vi "TCP Router Worker.vi"(7 "Name(\"\" to use uuid)":string="CSM-Module") -> ()   [LabVIEW 2020]
uses:
  <userlib>/_NEVSTOP/Communicable State Machine(CSM)/_Support/Priority Queue/Priority Queue.lvclass/Priority Queue.ctl
  4e85c3fb-ef85-4e26-a42c-c5beb394b70a.vi
  3806dceb-3f37-4f57-9f18-971811feca89.vi
  9016553c-cc0c-45c9-a77e-ad45dca8b9f9.vi
  29aca12e-f851-4e59-a4c5-05d041862115.vi
  20f56057-ddbc-4e16-b502-c2d75e71b705.vi
  <userlib>/_NEVSTOP/Communicable State Machine(CSM)/_Support/Process/CSMP-Async Call.vi
  <userlib>/_NEVSTOP/Communicable State Machine(CSM)/_Support/GlobalEvent/GEvt-Generate Status Log.vi
  <userlib>/_NEVSTOP/Communicable State Machine(CSM)/_Support/Process/CSMP-Broadcast.vi
  <userlib>/_NEVSTOP/Communicable State Machine(CSM)/_Support/GlobalEvent/GEvt-Generate Interrupt Log.vi
  <userlib>/_NEVSTOP/Communicable State Machine(CSM)/_Support/Process/CSMP-Register Status.vi
  <userlib>/_NEVSTOP/Communicable State Machine(CSM)/_Support/GlobalEvent/GEvt-Generate Register Log.vi
  <userlib>/_NEVSTOP/Communicable State Machine(CSM)/_Support/Process/CSMP-Unregister Status.vi
  <userlib>/_NEVSTOP/Communicable State Machine(CSM)/_Support/GlobalEvent/GEvt-Generate Unregister Log.vi
  <userlib>/_NEVSTOP/Communicable State Machine(CSM)/_Support/Process/CSMP-Sync Call.vi
  <userlib>/_NEVSTOP/Communicable State Machine(CSM)/_Support/CSMQ/_CSMObj-Unlock.vi
  <userlib>/_NEVSTOP/Communicable State Machine(CSM)/_Support/Process/CSMP-PostPostMsg.vi
  <userlib>/_NEVSTOP/Communicable State Machine(CSM)/_Support/Process/CSMP-PostSendMsg.vi
  <userlib>/_NEVSTOP/Communicable State Machine(CSM)/_Support/CSMQ/_CSMObj-Lock State.vi
  <userlib>/_NEVSTOP/Communicable State Machine(CSM)/_Support/Common/Splite Reason String Part.vi
  <userlib>/_NEVSTOP/Communicable State Machine(CSM)/_Support/Common/Trim Single line Text.vi
  <userlib>/_NEVSTOP/Communicable State Machine(CSM)/_Support/CSMQ/_CSMOFGV Release.vi
  <userlib>/_NEVSTOP/Communicable State Machine(CSM)/_Support/Common/Remove Comments from Line.vi
  <userlib>/_NEVSTOP/Communicable State Machine(CSM)/_Support/Common/Splite Single-line Message.vi
  <userlib>/_NEVSTOP/Communicable State Machine(CSM)/_Support/Common/Parse Next Single-line State.vi
  <userlib>/_NEVSTOP/Communicable State Machine(CSM)/_Support/CSMQ/_CSMOFGV Dequeue.vi
  <userlib>/_NEVSTOP/Communicable State Machine(CSM)/_Support/CSMQ/_CSMObj-Log Error if in a Remote Session.vi
  <userlib>/_NEVSTOP/Communicable State Machine(CSM)/_Support/GlobalEvent/GEvt-Generate State Change Log.vi
  <userlib>/_NEVSTOP/Communicable State Machine(CSM)/_Support/GlobalEvent/GEvt-Generate Remaining States Log.vi
  <userlib>/_NEVSTOP/Communicable State Machine(CSM)/_Support/GlobalEvent/GEvt-Generate Module Destroyed Log.vi
  <userlib>/_NEVSTOP/Communicable State Machine(CSM)/_Support/GlobalEvent/GEvt-Generate Complete Log.vi
  <userlib>/_NEVSTOP/Communicable State Machine(CSM)/_Support/GlobalEvent/GEvt-Generate Module Created Log.vi
  <userlib>/_NEVSTOP/Communicable State Machine(CSM)/_Support/GlobalEvent/Cache-GEvt Filter Object.vi
  <userlib>/_NEVSTOP/Communicable State Machine(CSM)/AdvanceAPI/CSM - Revert Arguments-Safe String.vi
  <userlib>/_NEVSTOP/Communicable State Machine(CSM)/AdvanceAPI/CSM - Make String Arguments Safe.vi
  <userlib>/_NEVSTOP/Communicable State Machine(CSM)/AdvanceAPI/CSM - Break Down Multiple States String.vi
  <userlib>/_NEVSTOP/Communicable State Machine(CSM)/AdvanceAPI/CSM - Compact Multiple States.vi
  <userlib>/_NEVSTOP/Communicable State Machine(CSM)/addons/API-String-Arugments-Support/_Support/Query Data as API String Arguments(variant).vi
  <userlib>/_NEVSTOP/Communicable State Machine(CSM)/_Support/CSMQ/_Obtain CSM Data Queue.vi
  <userlib>/_NEVSTOP/Communicable State Machine(CSM)/_Support/Priority Queue/Release Priority Queue.vi
  <userlib>/_NEVSTOP/Communicable State Machine(CSM)/_Support/CSMQ/_CSMObj-Message Check.vi
  <userlib>/_NEVSTOP/Communicable State Machine(CSM)/_Support/CSMQ/_CSMObj-Enqueue Cross-Module Message.vi
  <userlib>/_NEVSTOP/Communicable State Machine(CSM)/_Support/CSMQ/_CSMOFGV Get.vi
  <userlib>/_NEVSTOP/Communicable State Machine(CSM)/_Support/GlobalEvent/GEvt-Generate with Rule Check.vi
  <userlib>/_NEVSTOP/Communicable State Machine(CSM)/_Support/FGV-BroadcastRegistry/Cache-Broadcast Registry Search Result.vi
  <userlib>/_NEVSTOP/Communicable State Machine(CSM)/_Support/Common/Hex Str to U8 Data.vi
  <userlib>/_NEVSTOP/Communicable State Machine(CSM)/_Support/Common/Concatenate State with Arguments.vi
  <userlib>/_NEVSTOP/Communicable State Machine(CSM)/_Support/Common/U8 Data to Hex Str.vi
  <userlib>/_NEVSTOP/Communicable State Machine(CSM)/_Support/Priority Queue/Dequeue Element.vi
  <userlib>/_NEVSTOP/Communicable State Machine(CSM)/AdvanceAPI/CSM - Keywords.vi
  <userlib>/_NEVSTOP/Communicable State Machine(CSM)/_Support/Priority Queue/Obtain Priority Queue.vi
  <userlib>/_NEVSTOP/Communicable State Machine(CSM)/_Support/Priority Queue/Enqueue Element.vi
  <userlib>/_NEVSTOP/Communicable State Machine(CSM)/Utility/Trim Both Whitespace.vi
  <userlib>/_NEVSTOP/Communicable State Machine(CSM)/_Support/GlobalEvent/FGV-GlobalEventRef.vi
  <userlib>/_NEVSTOP/Communicable State Machine(CSM)/_Support/GlobalEvent/global-GEvnt Filter Change Flag.vi
  <userlib>/_NEVSTOP/Communicable State Machine(CSM)/_Support/GlobalEvent/FGV-GEvt Filter Obj.vi
  <userlib>/_NEVSTOP/Communicable State Machine(CSM)/_Support/CSMQ/_CSMOFGV Obtain.vi
  <userlib>/_NEVSTOP/Communicable State Machine(CSM)/_Support/GlobalEvent/LogFilter/LogFilter - Check.vi
  <userlib>/_NEVSTOP/Communicable State Machine(CSM)/Utility/Build Internal State String.vi
  <userlib>/_NEVSTOP/Communicable State Machine(CSM)/_Support/CSMQ/_CSMOFGV.vi
  <userlib>/_NEVSTOP/Communicable State Machine(CSM)/_Support/Error/CSM Not Allowed Message.vi
  <userlib>/_NEVSTOP/Communicable State Machine(CSM)/_Support/GlobalEvent/FGV-StatusChangeEventRef.vi
  <userlib>/_NEVSTOP/Communicable State Machine(CSM)/_Support/FGV-BroadcastRegistry/global-CSMQ FGV Change Flag.vi
  <userlib>/_NEVSTOP/Communicable State Machine(CSM)/_Support/FGV-BroadcastRegistry/global-Broadcast Cache Change Flag.vi
  <userlib>/_NEVSTOP/Communicable State Machine(CSM)/_Support/BroadcastRegistry/HelperVI/Broadcast Item Key.vi
  <userlib>/_NEVSTOP/Communicable State Machine(CSM)/_Support/FGV-BroadcastRegistry/FGV-BroadcastRegistry.vi
  <userlib>/_NEVSTOP/Communicable State Machine(CSM)/_Support/Message/Parse Register Message.vi
  <userlib>/_NEVSTOP/Communicable State Machine(CSM)/_Support/CSMQ/_CSMObj-Add Internal Registry Rule.vi
  <userlib>/_NEVSTOP/Communicable State Machine(CSM)/_Support/Message/Parse Unregister Message.vi
  <userlib>/_NEVSTOP/Communicable State Machine(CSM)/_Support/CSMQ/_CSMObj-Unregister Internal Registry Rules.vi
  <userlib>/_NEVSTOP/Communicable State Machine(CSM)/addons/API-String-Arugments-Support/_Support/Data To SingleElementsArray_with_itself_csm.vi
  <userlib>/_NEVSTOP/Communicable State Machine(CSM)/addons/API-String-Arugments-Support/_Support/Data To API String Arguments.vi
  <userlib>/_NEVSTOP/Communicable State Machine(CSM)/addons/API-String-Arugments-Support/_Support/Convert API String Arguments to Data(variant).vi
  <userlib>/_NEVSTOP/Communicable State Machine(CSM)/_Support/Error/CSM No Target Error.vi
  <userlib>/_NEVSTOP/Communicable State Machine(CSM)/_Support/Priority Queue/Priority Queue.lvclass
  <userlib>/_NEVSTOP/Communicable State Machine(CSM)/Communicable State Machine.lvlib
  <userlib>/_NEVSTOP/Communicable State Machine(CSM)/_csmHelper/API with lvcsm Support/CSM-Helper API with lvcsm Support.lvlib
panel:
  out "Error Occurred":errorcluster
  out "State History":string
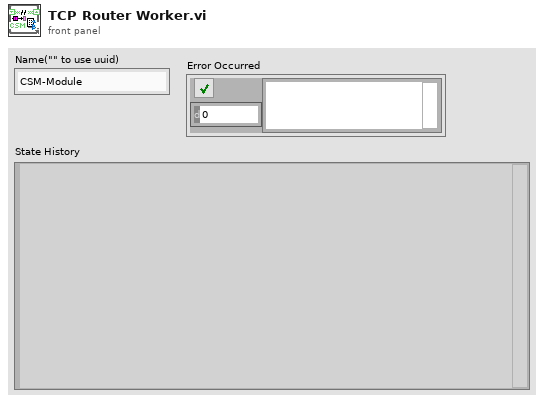
[diagram p1: front panel]
types:
  T1 = enum32{"Invalid", "Standard", "Closed", "Hidden", "Minimized", "Maximized"}
  T2 = enum32{"invalid app kind", "Development System", "Run Time System", "Student Edition", "Embedded LabVIEW", "Evaluation", "Custom"}
  T3 = typedef "Communicable State Machine.lvlib/_CSM_Response Source Message.ctl" = cluster{"‘State":string, "’Arguments":string, "’Error":errorcluster}
  T4 = cluster{"Current VI Reference":refnum<vi>, "Close Panel on Exit?":bool}
  T5 = cluster{"Core":cluster{"Current VI Reference":refnum<vi>, "Close Panel on Exit?":bool}, "Your Boolean data":bool, "Your string data":string}
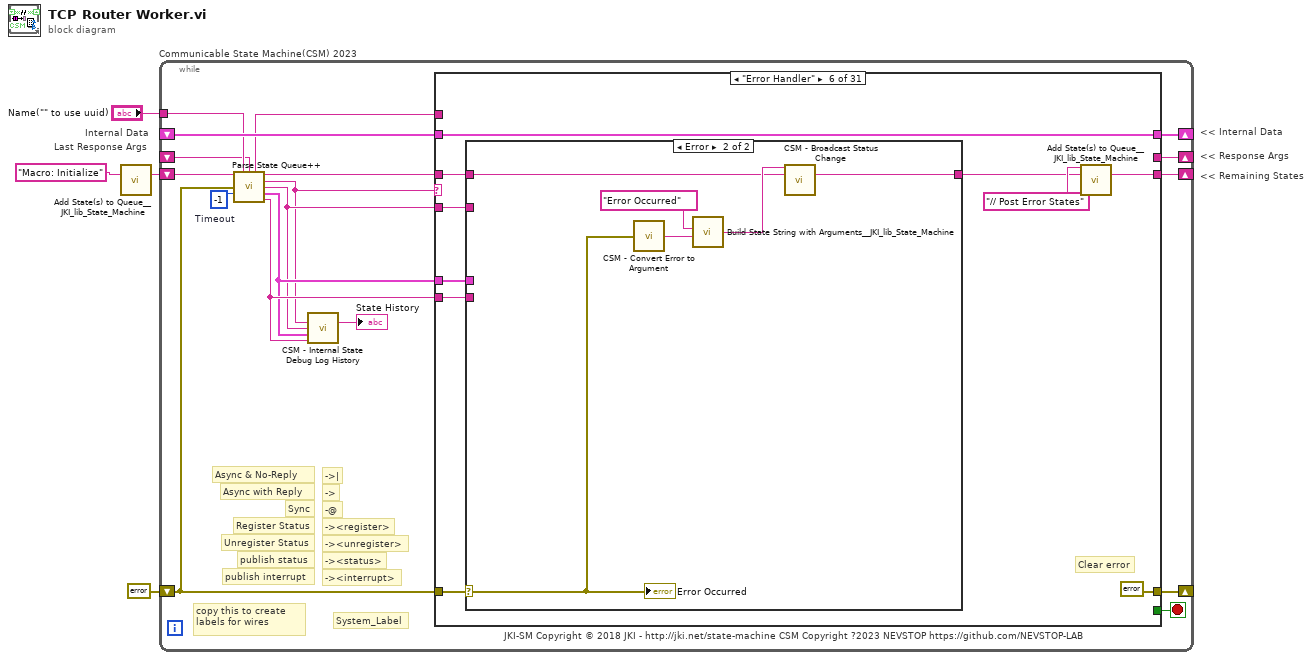
[diagram p0: block diagram]
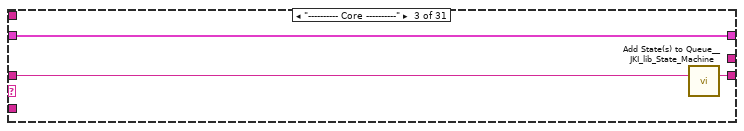
[diagram p4: hidden frame]
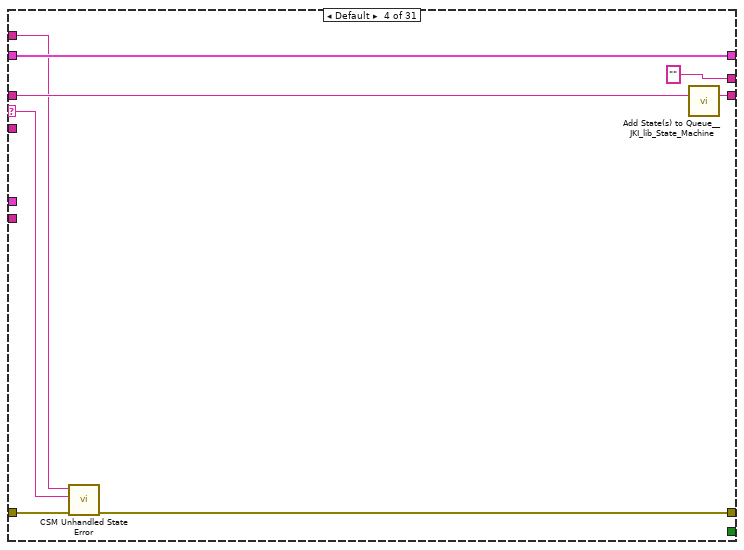
[diagram p5: hidden frame]
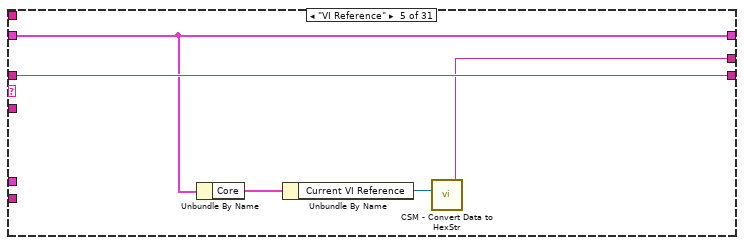
[diagram p6: hidden frame]
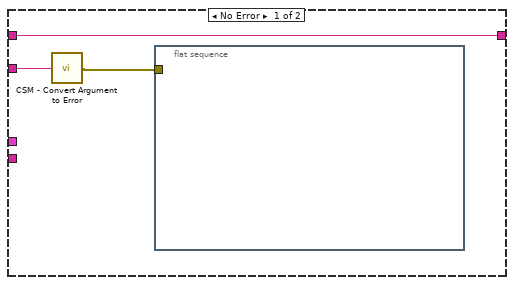
[diagram p7: hidden frame]
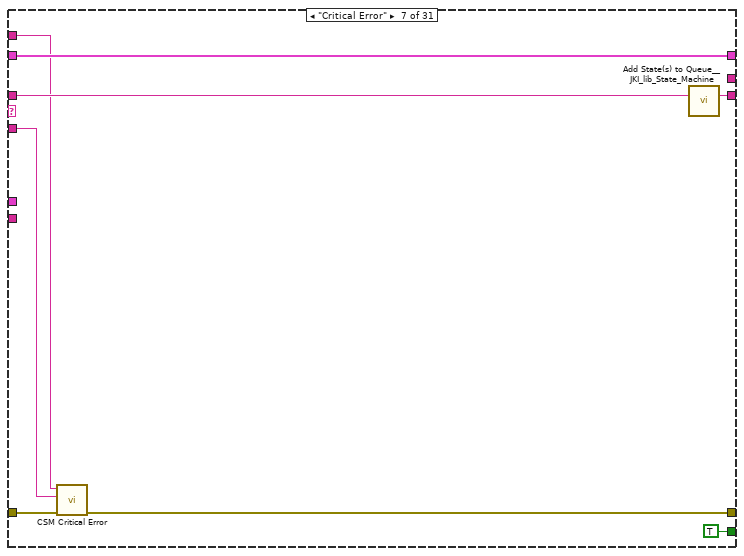
[diagram p8: hidden frame]
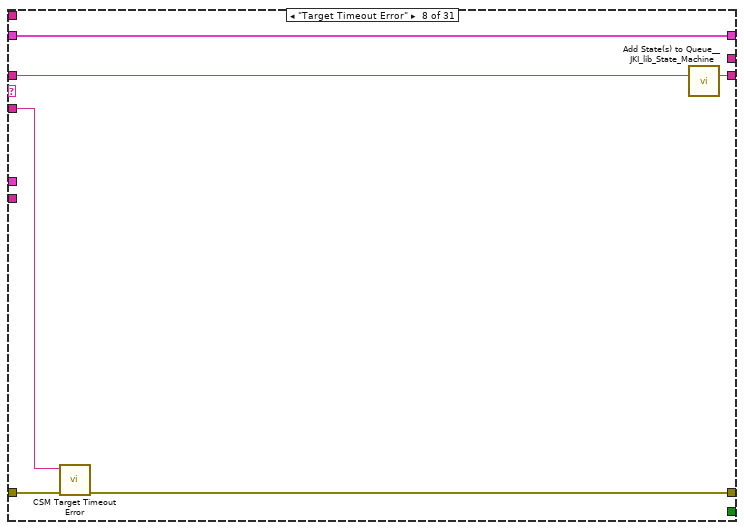
[diagram p9: hidden frame]
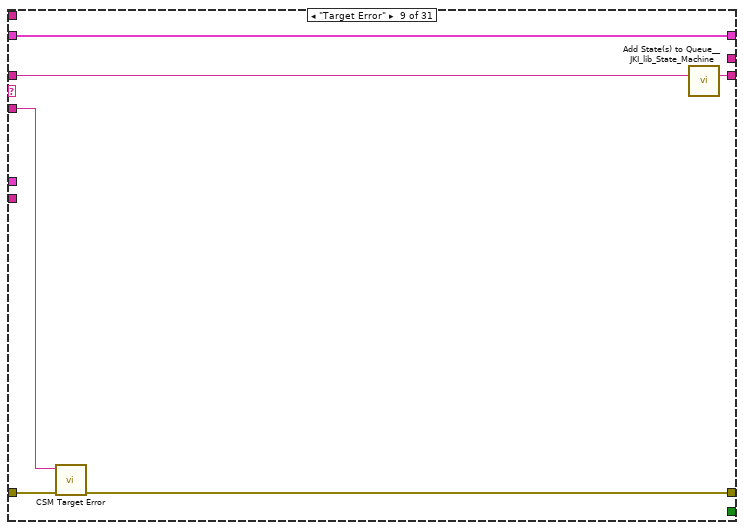
[diagram p10: hidden frame]
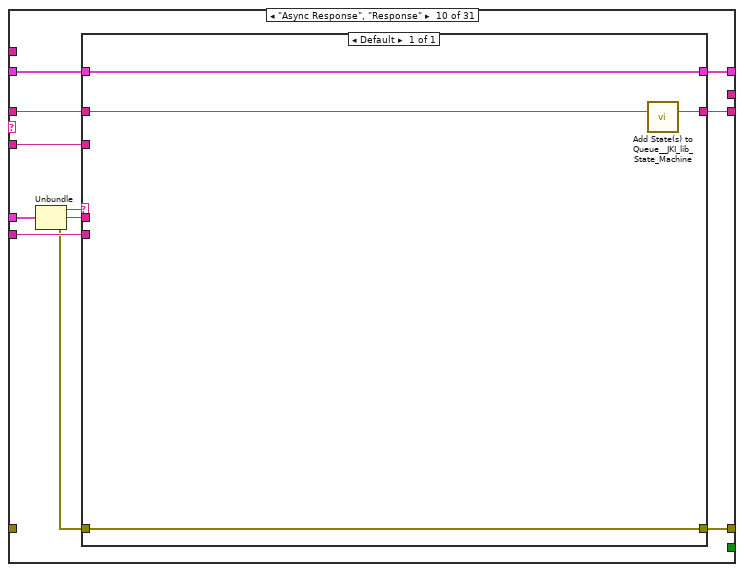
[diagram p11: hidden frame]
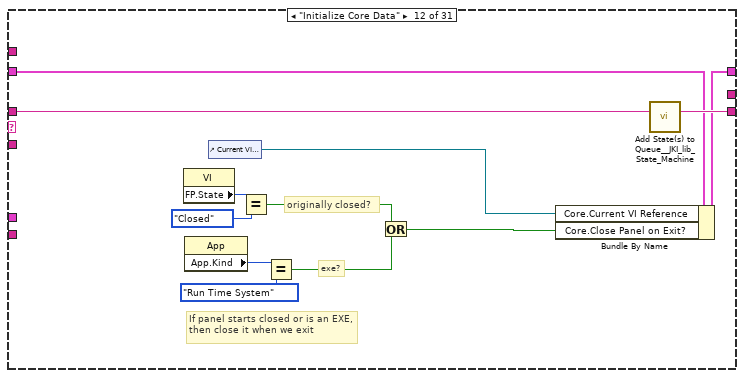
[diagram p13: hidden frame]
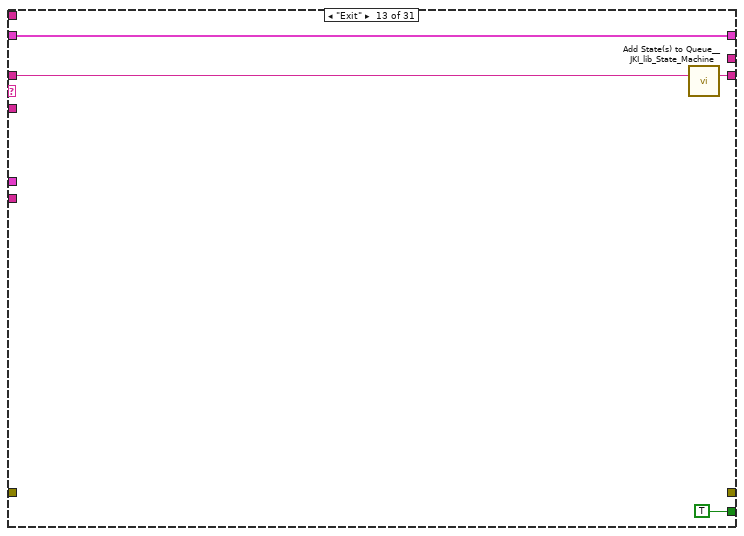
[diagram p14: hidden frame]
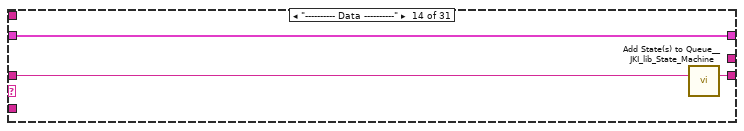
[diagram p15: hidden frame]
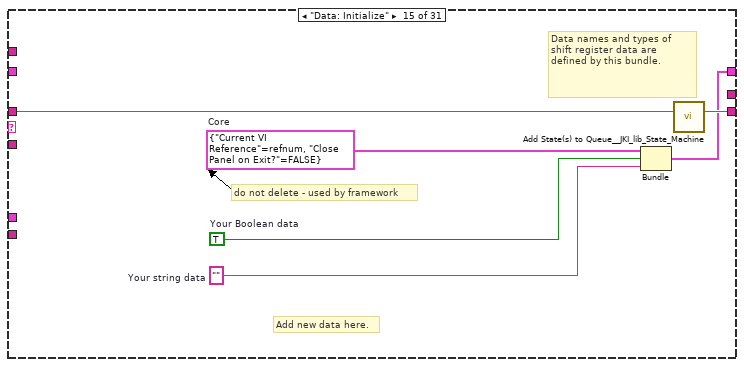
[diagram p16: hidden frame]
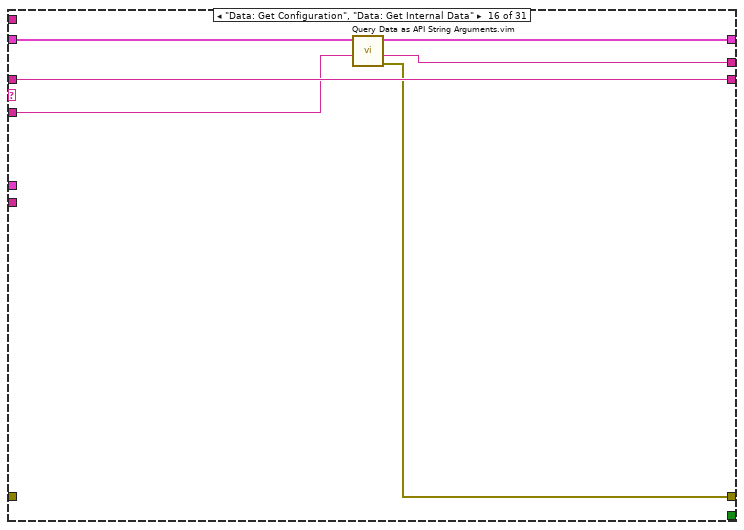
[diagram p17: hidden frame]
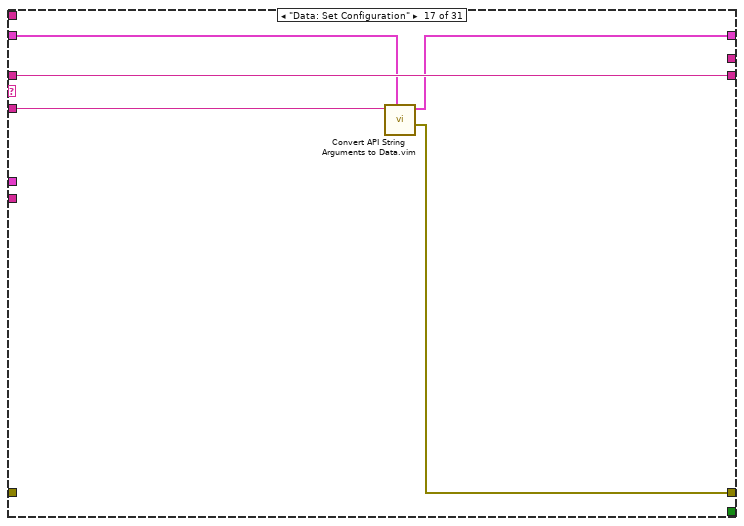
[diagram p18: hidden frame]
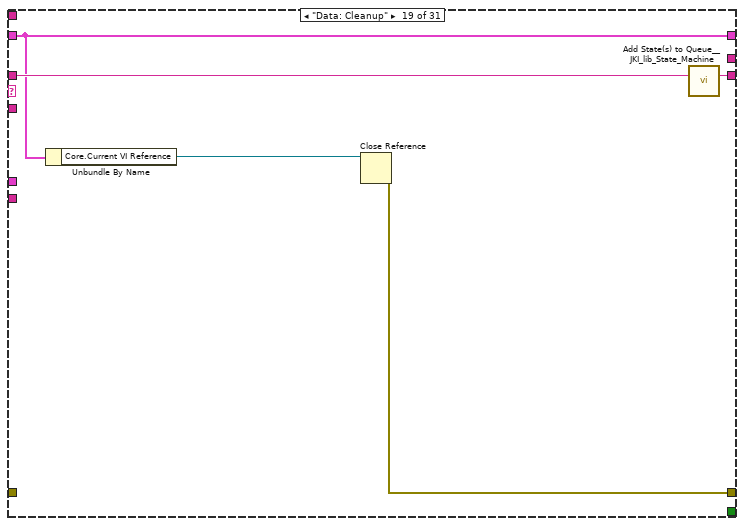
[diagram p20: hidden frame]
diagram:
  # "Last Response Args"
  # "Internal Data"
  # "<< Internal Data"
  # "<< Response Args"
  # "<< Remaining States"
  n1 = call <vilib>:"Add State(s) to Queue__JKI_lib_State_Machine.vi"("State(s) in (\"\")"="Macro: Initialize" ("Init States(\"Macro: Initialize\")")) -> ("States Out"=w2:string)  [unwired: 14 in]
  n2 = while "Communicable State Machine(CSM) 2023" {
    shift-right: [w17] -> _
    shift-left: _ -> [w16]
    shift-right: [w20] -> _
    shift-left: errorcluster {"status"=FALSE, "code"=0, "source"=""} ("error out") -> [w6]
    shift-right: [w19] -> _
    shift-left: w2 -> [w21]
    tunnel: "Name(\"\" to use uuid)" -> [w13]
    shift-right: [w14] -> _
    shift-left: _ -> [w8]
    stop <- w18 stop-if-true
    w15 = -1  # Timeout
    # "copy this to create labels for wires"
    # "System_Label"
    # "-><interrupt>"
    # "-><status>"
    # "-><unregister>"
    # "-><register>"
    # "-@"
    # "->"
    # "->|"
    # "publish interrupt"
    # "publish status"
    # "Unregister Status"
    # "Register Status"
    # "Sync"
    # "Async with Reply"
    # "Async & No-Reply"
    # "JKI-SM Copyright © 2018 JKI - http://jki.net/state-machine CSM Copyright ?2023 NEVSTOP https://github.com/NEVSTOP-LAB"
    n3 = call <userlib>:"Parse State Queue++.vi"("State Queue"=w21, "Name(\"\" to use uuid)"=w13, "Response Arguments"=w8, "Previous Error"=w6, "Dequeue Timeout(0ms)"=w15) -> ("Name Used"=w7:string, "Remaining States"=w22:string, "Current State"=w9:string, "Arguments"=w10:string, ">> Response Source Message >>"=w11:T3, ">> Source CSM >>"=w12:string)  [unwired: 5 in]
    n4 = call <userlib>:"CSM - Internal State Debug Log History.vi"("State"=w9, "Arguments (\"\")"=w10, ">> Response Source Message >>"=w11, "Source (\"\")"=w12) -> ("Debug Log"=→"State History":string)  [unwired: 11 in]
    n5 = case shown="\"Error Handler\"" w9 {
      selector: w9 -> [_ _ _ w32 _ _ _ _ _ _ _ _ _ _ _ _ _ _ _ _ _ _ _ _ _ _ _ _ _ _ _]
      tunnel: w22 -> [w23 w26 w29 w35 w42 w46 w68 w74 w80 w86 w98 w110 w114 w117 w123 w129 w134 w136 w141 w144 w148 w152 w154 w163 w182 w201 w220 w231 w236 w240 w243]
      tunnel: w10 -> [_ _ _ _ _ w45 w62 w71 w77 w85 _ _ _ _ _ w124 w133 _ _ _ _ _ _ w158 w177 w196 _ w229 _ _ _]
      tunnel: w16 -> [w24 w25 w27 w33 w39 w51 w66 w72 w78 w87 w97 w104 w112 w115 _ w128 w132 w135 w137 w142 w146 w150 w153 w162 w181 w200 w219 w230 w234 w238 w241]
      tunnel: [_ _ _ w37 _ errorcluster {"status"=FALSE, "code"=0, "source"=""} ("error out") w69 w70 w76 w90 _ _ _ _ _ w125 w130 _ w138 _ _ _ _ w156 w176 w195 w214 _ _ _ _] -> w20
      tunnel: w6 -> [_ _ _ w36 _ w49 w64 w75 w81 _ _ _ _ _ _ _ _ _ _ _ _ _ _ _ _ _ _ _ _ _ _]
      tunnel: [w23 w26 w28 w34 w42 w47 w67 w73 w79 w88 w98 w109 w113 w116 w122 w129 w134 w136 w140 w143 w147 w151 w154 w163 w182 w201 w220 w231 w235 w239 w242] -> w19
      tunnel: [_ _ _ _ _ _ TRUE _ _ _ _ _ TRUE _ _ _ _ _ _ _ _ _ _ _ _ _ _ _ _ _ _] -> w18
      tunnel: [w24 w25 w27 w33 w39 w51 w66 w72 w78 w89 w97 w108 w112 w115 w121 w127 w131 w135 w137 w142 w146 w150 w153 w162 w181 w200 w219 w230 w234 w238 w241] -> w17
      tunnel: w12 -> [_ _ _ _ _ w44 _ _ _ w83 _ _ _ _ _ _ _ _ _ _ _ _ _ _ _ _ _ _ _ _ _]
      tunnel: w11 -> [_ _ _ _ _ w43 _ _ _ w84 _ _ _ _ _ _ _ _ _ _ _ _ _ _ _ _ _ _ _ _ _]
      tunnel: [_ _ _ "" w38 _ _ _ _ _ _ _ _ _ _ w126 _ _ _ _ _ _ _ w155 w174 w194 _ w228 _ "Action Finished" _] -> w14
      tunnel: w7 -> [_ _ _ w30 _ _ w63 _ _ _ _ _ _ _ _ _ _ _ _ _ _ _ _ w157 w175 w193 w215 _ _ _ _]
      frame "", "Idle" {
      }
      frame "CSM Documentation" {
      }
      frame "---------- Core ----------" {
        n6 = call <vilib>:"Add State(s) to Queue__JKI_lib_State_Machine.vi"("State(s) in (\"\")"=w29) -> ("States Out"=w28:string)  [unwired: 14 in]
      }
      frame Default {
        n7 = call <userlib>:"CSM Unhandled State Error.vi"("error in (no error)"=w36, "Current State"=w32, "CSM Name"=w30) -> ("error out"=w37:errorcluster)  [unwired: 8 in]
        n8 = call <vilib>:"Add State(s) to Queue__JKI_lib_State_Machine.vi"("State(s) in (\"\")"=w35) -> ("States Out"=w34:string)  [unwired: 14 in]
      }
      frame "VI Reference" {
        n9 = Unbundle By Name(w39) -> ("Core"=w41:T4)
        n10 = Unbundle By Name(w41) -> ("Current VI Reference"=w40:refnum<vi>)
        n11 = call <userlib>:"CSM - Convert Data to HexStr.vi"("Variant"=w40) -> ("HEX String (0-9,A-F)"=w38:string)  [unwired: 8 in]
      }
      frame "Error Handler" {
        # "Clear error"
        n12 = case shown="Error" w49 {
          selector: w49 -> [_ w56]
          tunnel: [w55 w58] -> w48
          tunnel: w46 -> [w55 w57]
          tunnel: w45 -> [w54 _]
          tunnel: w44 -> [_ _]
          tunnel: w43 -> [_ _]
          frame No Error {
            n13 = call <userlib>:"CSM - Convert Argument to Error.vi"("Argument"=w54) -> ("error"=w53:errorcluster)  [unwired: 4 in]
            n14 = flat-sequence {
              tunnel: w53 -> [_]
              frame #0 {
              }
            }
          }
          frame Error {
            n15 = call <userlib>:"CSM - Convert Error to Argument.vi"("error"=w56) -> ("Argument"=w60:string)  [unwired: 4 in]
            n16 = call <vilib>:"Build State String with Arguments__JKI_lib_State_Machine.vi"("Arguments (\"\")"=w60, "State"="Error Occurred" ("Status with Arguments")) -> ("State with Arguments"=w59:string)  [unwired: 4 in]
            n17 = call <userlib>:"CSM - Broadcast Status Change.vi"("Status with Arguments"=w59, "State Queue"=w57) -> ("Remaining States"=w58:string)  [unwired: 13 in]
            "Error Occurred" <- w56
          }
        }
        n18 = call <vilib>:"Add State(s) to Queue__JKI_lib_State_Machine.vi"("State(s) in Front (\"\")"="// Post Error States", "State(s) in (\"\")"=w48) -> ("States Out"=w47:string)  [unwired: 13 in]
      }
      frame "Critical Error" {
        n19 = call <userlib>:"CSM Critical Error.vi"("error in (no error)"=w64, "Arugments(as Reason)"=w62, "CSM Name"=w63) -> ("error out"=w69:errorcluster)  [unwired: 8 in]
        n20 = call <vilib>:"Add State(s) to Queue__JKI_lib_State_Machine.vi"("State(s) in (\"\")"=w68) -> ("States Out"=w67:string)  [unwired: 14 in]
      }
      frame "Target Timeout Error" {
        n21 = call <userlib>:"CSM Target Timeout Error.vi"("error in (no error)"=w75, "Arguments(as CSM Name)"=w71) -> ("error out"=w70:errorcluster)  [unwired: 9 in]
        n22 = call <vilib>:"Add State(s) to Queue__JKI_lib_State_Machine.vi"("State(s) in (\"\")"=w74) -> ("States Out"=w73:string)  [unwired: 14 in]
      }
      frame "Target Error" {
        n23 = call <userlib>:"CSM Target Error.vi"("error in (no error)"=w81, "Arguments(as CSM Name)"=w77) -> ("error out"=w76:errorcluster)  [unwired: 9 in]
        n24 = call <vilib>:"Add State(s) to Queue__JKI_lib_State_Machine.vi"("State(s) in (\"\")"=w80) -> ("States Out"=w79:string)  [unwired: 14 in]
      }
      frame "Async Response", "Response" {
        n25 = Unbundle(w84) -> ("‘State"=w92:string, "’Arguments"=w91:string, "’Error"=w82:errorcluster)
        n26 = case shown="Default" w92 {
          tunnel: [w93] -> w88
          tunnel: w86 -> [w94]
          tunnel: [w96] -> w89
          tunnel: w87 -> [w96]
          tunnel: [w95] -> w90
          tunnel: w82 -> [w95]
          tunnel: w83 -> [_]
          tunnel: w85 -> [_]
          tunnel: w91 -> [_]
          frame Default {
            n27 = call <vilib>:"Add State(s) to Queue__JKI_lib_State_Machine.vi"("State(s) in (\"\")"=w94) -> ("States Out"=w93:string)  [unwired: 14 in]
          }
        }
      }
      frame "Async Message Posted" {
      }
      frame "Initialize Core Data" {
        # "originally closed?"
        # "exe?"
        # "If panel starts closed or is an EXE, then close it when we exit"
        n28 = property class="VI"() -> ("FP.State"=w101:T1)  [unwired: 2 in, 2 out]
        n29 = property class="App"() -> ("App.Kind"=w107:T2)  [unwired: 2 in, 2 out]
        n30 = control-ref of="Current VI Reference"() -> (w102:refnum<vi>)
        n31 = Equal?(x=w101, y=T1."Closed" ("Front Panel Window:State")) -> (x = y?=w99:bool)
        n32 = Equal?(x=w107, y=T2."Run Time System" ("Application:Kind")) -> (x = y?=w105:bool)
        n33 = Or(x=w99, y=w105) -> (x .or. y?=w103:bool)
        n34 = Bundle By Name(cluster=w104, "Core.Current VI Reference"=w102, "Core.Close Panel on Exit?"=w103) -> (w108:T5)
        n35 = call <vilib>:"Add State(s) to Queue__JKI_lib_State_Machine.vi"("State(s) in (\"\")"=w110) -> ("States Out"=w109:string)  [unwired: 14 in]
      }
      frame "Exit" {
        n36 = call <vilib>:"Add State(s) to Queue__JKI_lib_State_Machine.vi"("State(s) in (\"\")"=w114) -> ("States Out"=w113:string)  [unwired: 14 in]
      }
      frame "---------- Data ----------" {
        n37 = call <vilib>:"Add State(s) to Queue__JKI_lib_State_Machine.vi"("State(s) in (\"\")"=w117) -> ("States Out"=w116:string)  [unwired: 14 in]
      }
      frame "Data: Initialize" {
        w118 = T4 {"Current VI Reference"=refnum, "Close Panel on Exit?"=FALSE}  # Core
        w120 = TRUE  # Your Boolean data
        w119 = ""  # Your string data
        # "do not delete - used by framework"
        # "Add new data here."
        # "Data names and types of shift register data are defined by this bundle."
        n38 = Bundle("Core"=w118, "Your Boolean data"=w120, "Your string data"=w119) -> (w121:T5)  [unwired: 1 in]
        n39 = call <vilib>:"Add State(s) to Queue__JKI_lib_State_Machine.vi"("State(s) in (\"\")"=w123) -> ("States Out"=w122:string)  [unwired: 14 in]
      }
      frame "Data: Get Configuration", "Data: Get Internal Data" {
        n40 = call "Query Data as API String Arguments.vim"("Setting Name"=w124, "Internal Data"=w128) -> ("error"=w125:errorcluster, "Setting as String"=w126:string, "Internal Data(dup)"=w127:T5)  [unwired: 7 in]
      }
      frame "Data: Set Configuration" {
        n41 = call "Convert API String Arguments to Data.vim"("Type"=w132, "String"=w133) -> ("error"=w130:errorcluster, "Data"=w131:T5)  [unwired: 6 in]
      }
      frame "Data: Update Indicators" {
      }
      frame "Data: Cleanup" {
        n42 = Unbundle By Name(w137) -> ("Core.Current VI Reference"=w139:refnum<vi>)
        n43 = Close Reference(reference=w139) -> (error out=w138:errorcluster)  [unwired: 1 in]
        n44 = call <vilib>:"Add State(s) to Queue__JKI_lib_State_Machine.vi"("State(s) in (\"\")"=w141) -> ("States Out"=w140:string)  [unwired: 14 in]
      }
      frame "---------- Macro ----------" {
        n45 = call <vilib>:"Add State(s) to Queue__JKI_lib_State_Machine.vi"("State(s) in (\"\")"=w144) -> ("States Out"=w143:string)  [unwired: 14 in]
      }
      frame "Macro: Initialize" {
        n46 = call <vilib>:"Add State(s) to Queue__JKI_lib_State_Machine.vi"("State(s) in Front (\"\")"="Data: Initialize\nInitialize Core Data\nData: Update Indicators", "State(s) in (\"\")"=w148) -> ("States Out"=w147:string)  [unwired: 13 in]
      }
      frame "Macro: Exit" {
        n47 = call <vilib>:"Add State(s) to Queue__JKI_lib_State_Machine.vi"("State(s) in Front (\"\")"="Data: Cleanup\nExit", "State(s) in (\"\")"=w152) -> ("States Out"=w151:string)  [unwired: 13 in]
      }
      frame "---------- API ----------" {
      }
      frame "list API", "list interface" {
        n48 = call <userlib>:"CSM - Check If Module Exists.vi"("CSM Name"=w158) -> ("Error out"=w161:errorcluster, "Exist?"=w159:bool, "CSM Name(dup)"=w160:string)  [unwired: 8 in]
        n49 = case shown="True" w159 {
          tunnel: [w165 _] -> w156
          tunnel: w161 -> [w170 _]
          tunnel: w160 -> [w169 w172]
          tunnel: w157 -> [w166 _]
          tunnel: [w164 w171] -> w155
          frame True {
            n50 = call <userlib>:"Read CSM API with lvcsm Support.vi"("Current Module(\"\" to generate a ID)"=w166, "error in (no error)"=w170, "CSM Name"=w169) -> ("Error out"=w168:errorcluster, "CSMAPI List"=w167:string[])  [unwired: 7 in]
            n51 = call "Convert Data To API String Arguments.vim"("error in (no error)"=w168, "data"=w167) -> ("error out"=w165:errorcluster, "String"=w164:string)  [unwired: 6 in]
          }
          frame False {
            n52 = Format Into String(format string="\"%s\" module is not existing", w172) -> (resulting string=w171:string)  [unwired: 2 in, 1 out]
          }
        }
      }
      frame "List State", "List States" {
        n53 = call <userlib>:"CSM - Check If Module Exists.vi"("CSM Name"=w177) -> ("Error out"=w180:errorcluster, "Exist?"=w178:bool, "CSM Name(dup)"=w179:string)  [unwired: 8 in]
        n54 = case shown="False" w178 {
          tunnel: [w184 _] -> w176
          tunnel: w180 -> [w188 _]
          tunnel: w179 -> [w187 w191]
          tunnel: w175 -> [w185 _]
          tunnel: [w183 w190] -> w174
          frame True {
            n55 = call <userlib>:"Read CSM States with lvcsm Support.vi"("Current Module(\"\" to generate a ID)"=w185, "error in (no error)"=w188, "CSM Name"=w187) -> ("Error out"=w186:errorcluster, "CSMAPI List"=w189:string[])  [unwired: 7 in]
            n56 = call "Convert Data To API String Arguments.vim"("error in (no error)"=w186, "data"=w189) -> ("error out"=w184:errorcluster, "String"=w183:string)  [unwired: 6 in]
          }
          frame False {
            n57 = Format Into String(format string="\"%s\" module is not existing", w191) -> (resulting string=w190:string)  [unwired: 2 in, 1 out]
          }
        }
      }
      frame "help" {
        n58 = call <userlib>:"CSM - Check If Module Exists.vi"("CSM Name"=w196) -> ("Error out"=w199:errorcluster, "Exist?"=w197:bool, "CSM Name(dup)"=w198:string)  [unwired: 8 in]
        n59 = case shown="True" w197 {
          tunnel: [w204 _] -> w195
          tunnel: w199 -> [w210 _]
          tunnel: w198 -> [w209 w212]
          tunnel: [w203 w211] -> w194
          tunnel: w193 -> [w202 _]
          frame True {
            n60 = call <userlib>:"CSM - Module VI Reference.vi"("Current Module(\"\" to generate a ID)"=w202, "error in (no error)"=w210, "CSM Name"=w209) -> ("error out"=w208:errorcluster, "CSM Module VIRef"=w206:refnum<vi>)  [unwired: 7 in]
            n61 = property class="VI"(reference=w206, error in=w208) -> (error out=w207:errorcluster, "Description"=w205:string)  [unwired: 1 out]
            n62 = call "Convert Data To API String Arguments.vim"("error in (no error)"=w207, "data"=w205) -> ("error out"=w204:errorcluster, "String"=w203:string)  [unwired: 6 in]
          }
          frame False {
            n63 = Format Into String(format string="\"%s\" module is not existing", w212) -> (resulting string=w211:string)  [unwired: 2 in, 1 out]
          }
        }
      }
      frame "Refresh lvcsm" {
        n64 = call <userlib>:"CSM - List Modules.vi"() -> ("Error out"=w218:errorcluster, "Module Names"=w217:string[])  [unwired: 10 in]
        n65 = for {
          tunnel: w218 -> [w227]
          tunnel: w217 -> [w225] mode=indexing
          tunnel: [w222] -> w216 mode=indexing
          tunnel: w215 -> [w221]
          n66 = call <userlib>:"Read CSM States with lvcsm Support.vi"("Current Module(\"\" to generate a ID)"=w221, "error in (no error)"=w227, "Force?(F)"=TRUE, "CSM Name"=w225) -> ("Error out"=w226:errorcluster)  [unwired: 6 in, 1 out]
          n67 = call <userlib>:"Read CSM API with lvcsm Support.vi"("Current Module(\"\" to generate a ID)"=w221, "error in (no error)"=w226, "Force?(F)"=TRUE, "CSM Name"=w225) -> ("Error out"=w222:errorcluster)  [unwired: 6 in, 1 out]
        }
        n68 = Merge Errors(w216) -> (w214:errorcluster)
      }
      frame "API: API2" {
        # "unpack Hex String  to Variant\nif complex parameter is needed."
        n69 = call <userlib>:"CSM - Convert HexStr to Data.vi"("HEX String"=w229) -> ()  [unwired: 7 in, 2 out]
        n70 = disable-structure shown="Enabled" {
          disable-tunnel: [w232 "API2 Response"] -> w228
          frame Disabled {
            # "pack variant to hexstr \nif complex response is needed."
            # "complex Response"
            n71 = call <userlib>:"CSM - Convert Data to HexStr.vi"() -> ("HEX String (0-9,A-F)"=w232:string)  [unwired: 9 in]
          }
          frame Enabled {
          }
        }
      }
      frame "---------- Action ----------" {
        n72 = call <vilib>:"Add State(s) to Queue__JKI_lib_State_Machine.vi"("State(s) in (\"\")"=w236) -> ("States Out"=w235:string)  [unwired: 14 in]
      }
      frame "Action: Action1" {
        n73 = call <vilib>:"Add State(s) to Queue__JKI_lib_State_Machine.vi"("State(s) in (\"\")"=w240) -> ("States Out"=w239:string)  [unwired: 14 in]
      }
      frame "Action: Action2" {
        n74 = call <vilib>:"Add State(s) to Queue__JKI_lib_State_Machine.vi"("State(s) in (\"\")"=w243) -> ("States Out"=w242:string)  [unwired: 14 in]
      }
    }
  }
